vi "Global settings.vi"() -> ()   [LabVIEW 2018]
uses:
  <vilib>/Utility/miscctls.llb/LVDateTimeRec.ctl
  <vilib>/addons/database/Auxilliary.llb/DB Tools Format Datetime String (Time Stamp).vi
  <vilib>/lvdsc/NI_DSC.lvlib
  <vilib>/addons/database/NI_Database_API.lvlib
panel:
  in  "Clear":bool
  out "date time rec 4":T1
  out "x-y 2":T1
  out "Accident 2":bool
  out "Database Data":i32(listbox)=-1
  in  "Accident":bool
  in  "Traffic light failure":bool
  in  "Closesettings":bool
  in  "Set state":T2(ring)
  in  "State change":bool=TRUE
  in  "Time scale":dbl=1.0
  out "date time rec":T1
  out "x > y?":bool
  in  "Difference":dbl=5.0
  in  "Traffic volume 2":dbl(knob) scale=0.0..10.0
  in  "Traffic volume 1":dbl(knob) scale=0.0..10.0
  # "AUTO"
  # "MANUAL"
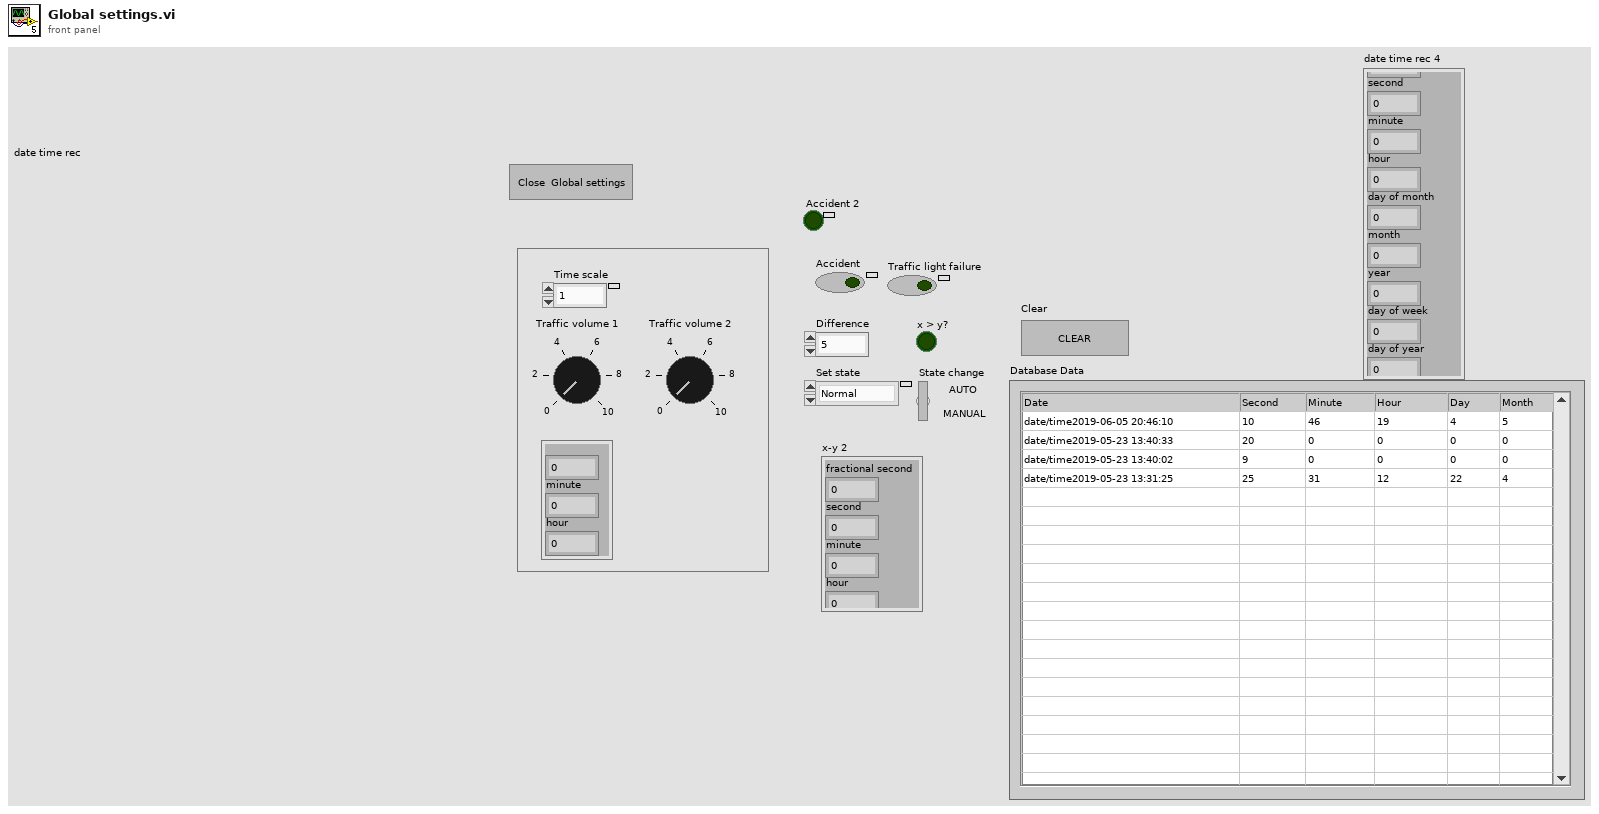
[diagram p1: front panel]
types:
  T1 = typedef "LVDateTimeRec.ctl" = cluster{"fractional second":dbl, "second":i32, "minute":i32, "hour":i32, "day of month":i32, "month":i32, "year":i32, "day of week":i32, "day of year":i32, "DST":i32}
  T2 = enum16{"Normal", "Night", "Traffic jam 1", "Traffic jam 2"}
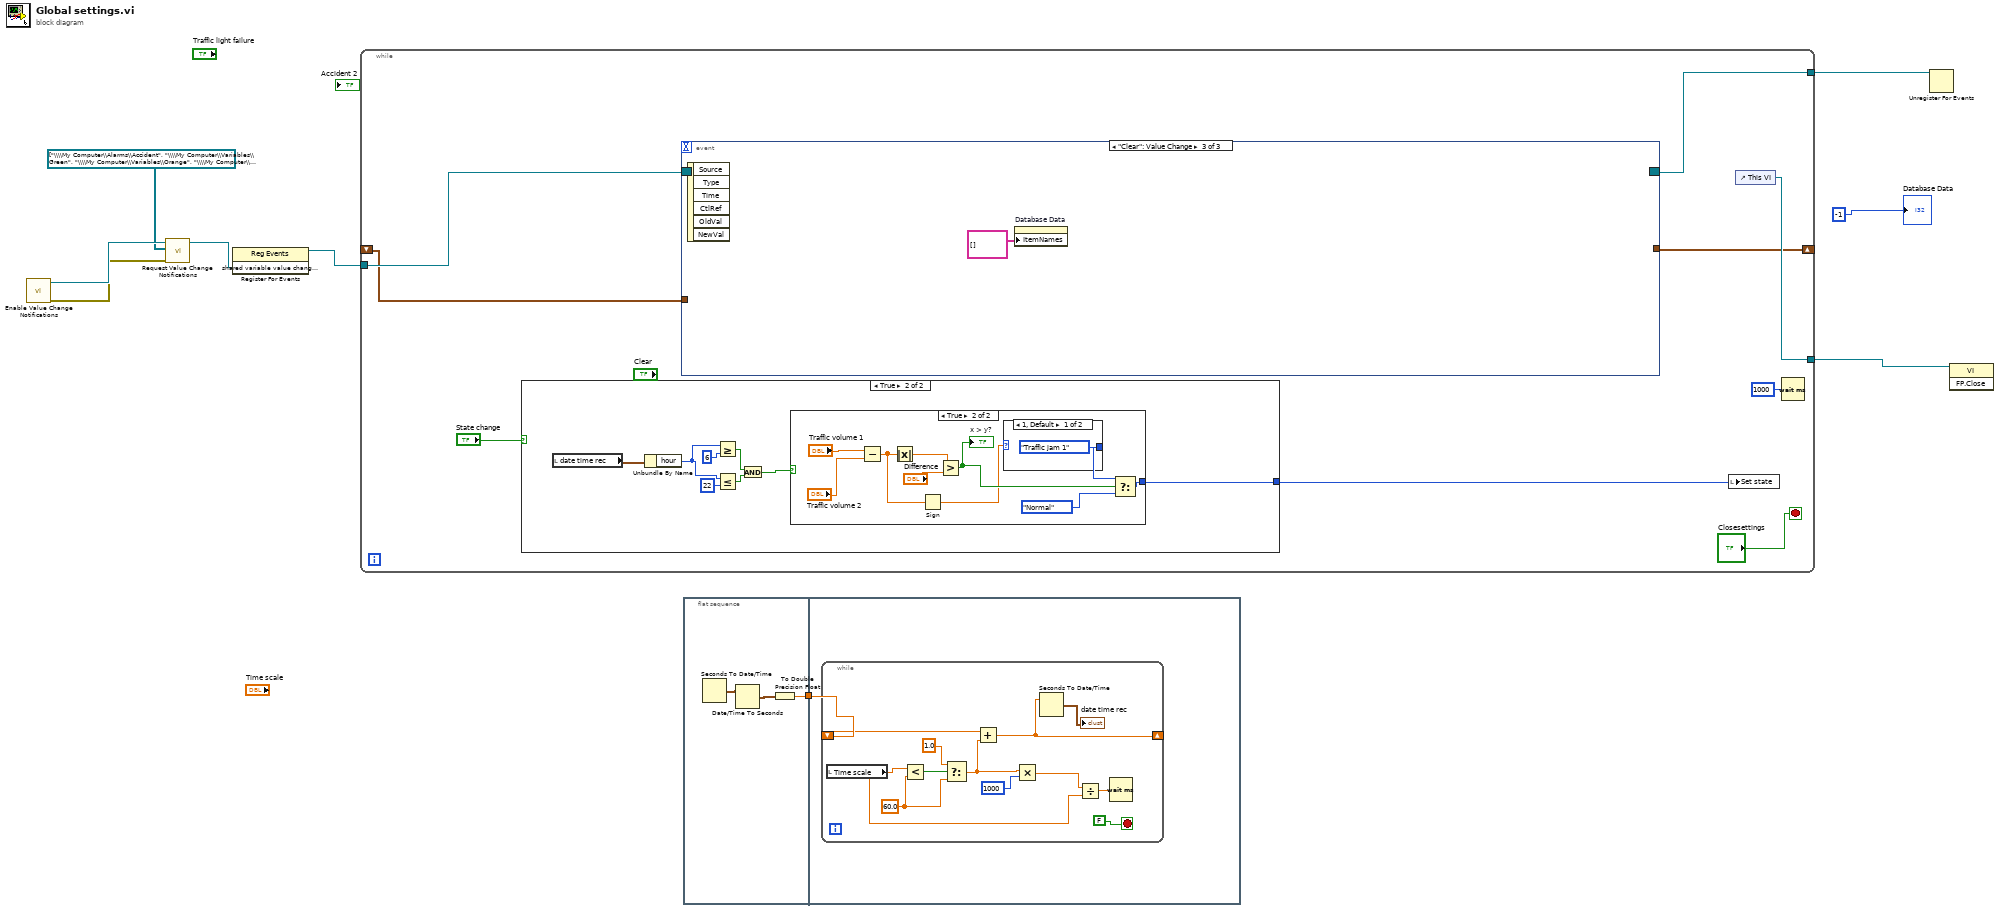
[diagram p0: block diagram]
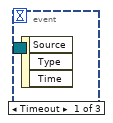
[diagram p2: hidden frame]
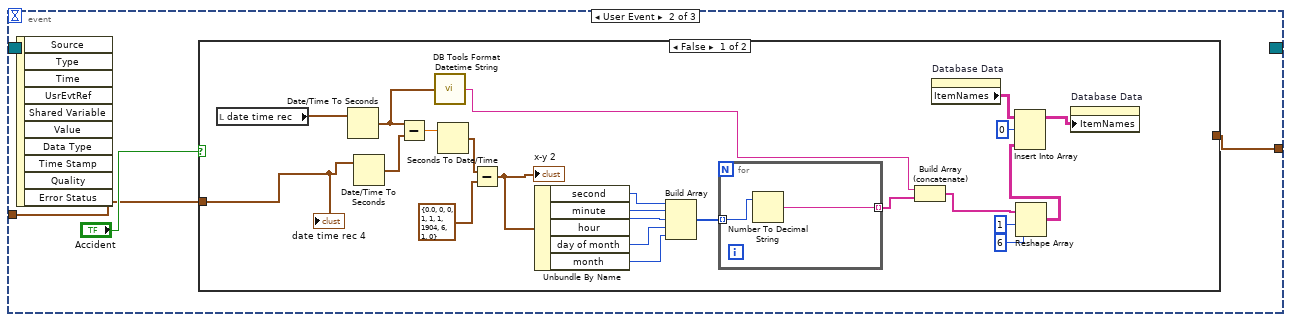
[diagram p3: hidden frame]
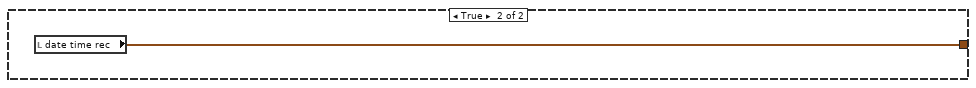
[diagram p4: hidden frame]
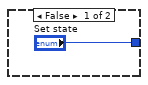
[diagram p5: hidden frame]
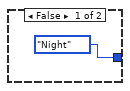
[diagram p6: hidden frame]
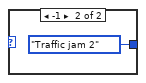
[diagram p7: hidden frame]
diagram:
  n1 = call <vilib>:"Enable Value Change Notifications.vi"() -> ("error out"=w4:errorcluster, "shared variable value change notification"=w5:refnum<user-event>)  [unwired: 1 in, 9 out]
  n2 = call <vilib>:"Request Value Change Notifications.vi"("error in (no error)"=w4, "shared variables"=refnum<k21>[] ["\\\\My Computer\\Alarms\\Accident", "\\\\My Computer\\Variables\\Green", "\\\\My Computer\\Variables\\Orange", "\\\\My Computer\\Variables\\Red", "\\\\My Computer\\Variables\\Yellow"], "notification refnum"=w5) -> ("shared variable value change notification"=w6:refnum<user-event>)  [unwired: 1 in, 7 out]
  n3 = register-events(w6) -> (reference out=w2:refnum<event-registration>)  [unwired: 2 in, 1 out]
  n4 = while {
    tunnel: [w15] -> w8
    tunnel: w2 -> [w13]
    tunnel: [w12] -> w1
    shift-right: [w11] -> _
    shift-left: _ -> [w10]
    stop <- "Closesettings" stop-if-true
    n5 = case shown="True" "State change" {
      tunnel: ["Set state" w50] -> w16
      frame False {
      }
      frame True {
        n6 = local read "date time rec"() -> (w57:T1)
        n7 = Unbundle By Name(w57) -> ("hour"=w51:i32)
        n8 = Greater Or Equal?(x=w51, y=6 ("x")) -> (x >= y?=w56:bool)
        n9 = Less Or Equal?(x=w51, y=22) -> (x <= y?=w54:bool)
        n10 = And(x=w56, y=w54) -> (x .and. y?=w53:bool)
        n11 = case shown="True" w53 {
          tunnel: [T2."Night" ("Set state") w61] -> w50
          frame False {
          }
          frame True {
            n12 = Subtract(x="Traffic volume 1", y="Traffic volume 2") -> (x-y=w63:dbl)
            n13 = Absolute Value(x=w63) -> (abs(x)=w66:dbl)
            n14 = Sign(1:w63) -> (0:w60:dbl)
            n15 = Greater?(x=w66, y="Difference") -> (0:w64:bool)
            "x > y?" <- w64
            n16 = case shown="1, Default" w60 {
              tunnel: [T2."Traffic jam 1" ("Set state") T2."Traffic jam 2" ("Set state")] -> w59
              frame 1, Default {
              }
              frame -1 {
              }
            }
            n17 = Select(t=w59, s=w64, f=T2."Normal" ("Set state")) -> (s? t:f=w61:T2)
          }
        }
      }
    }
    n18 = event shown="[2] \"Clear\": Value Change" {
      selector: w13 -> [_ _ _]
      dyn-events: [_ _ _] -> w12
      timeout: _ -> [_ _ _]
      tunnel: [_ w20 _] -> w11
      tunnel: w10 -> [_ w19 _]
      event Timeout {
        n19 = event-data() -> ()  [unwired: 1 in, 3 out]
      }
      event User Event {
        n20 = event-data() -> ()  [unwired: 1 in, 10 out]
        n21 = case shown="False" "Accident" {
          tunnel: [_ w47] -> w20
          tunnel: w19 -> [w39 _]
          frame False {
            n22 = local read "date time rec"() -> (w44:T1)
            n23 = Date/Time To Seconds(2:w44) -> (0:w25:timestamp)  [unwired: 1 in]
            n24 = Date/Time To Seconds(2:w39) -> (0:w43:timestamp)  [unwired: 1 in]
            n25 = Subtract(x=w25, y=w43) -> (x-y=w42:dbl)
            n26 = call-poly <vilib>:"DB Tools Format Datetime String.vi"("time stamp"=w25) -> ("date/time string"=w22:string)
            n27 = Seconds To Date/Time(time stamp (now)=w42) -> (date time rec=w41:T1)  [unwired: 1 in]
            n28 = Subtract(x=w41, y=T1 {"fractional second"=0.0, "second"=0, "minute"=0, "hour"=1, "day of month"=1, "month"=1, "year"=1904, "day of week"=6, "day of year"=1, "DST"=0} ("date time rec")) -> (x-y=w33:T1)
            "x-y 2" <- w33
            n29 = Unbundle By Name(w33) -> ("second"=w38:i32, "minute"=w37:i32, "hour"=w36:i32, "day of month"=w35:i32, "month"=w34:i32)
            n30 = Build Array(w38, w37, w36, w35, w34) -> (w32:i32[])
            n31 = for {
              tunnel: w32 -> [w46] mode=indexing
              tunnel: [w45] -> w24 mode=indexing
              n32 = Number To Decimal String(number=w46) -> (decimal integer string=w45:string)  [unwired: 1 in]
            }
            n33 = Build Array (concatenate)(w22, w24) -> (w23:string[])
            n34 = property on="Database Data" class="MCListbox (strict)"() -> ("ItemNames"=w29:string[][])  [unwired: 2 in, 2 out]
            n35 = Reshape Array "Reshape Array"(w23, 1 ("dimension size"), 6 ("dimension size")) -> (w28:string[][])
            n36 = Insert Into Array(array=w29, index (row)=0, new element=w28) -> (w27:string[][])  [unwired: 1 in]
            n37 = property on="Database Data" class="MCListbox (strict)"("ItemNames"=w27) -> ()  [unwired: 2 in, 2 out]
            "date time rec 4" <- w39
          }
          frame True {
            n38 = local read "date time rec"() -> (w47:T1)
          }
        }
      }
      event "Clear": Value Change {
        n39 = event-data() -> ()  [unwired: 1 in, 6 out]
        n40 = property on="Database Data" class="MCListbox (strict)"("ItemNames"=string[][] [] ("Item Names")) -> ()  [unwired: 2 in, 2 out]
      }
    }
    n41 = local write "Set state"(w16) -> ()
    n42 = control-ref of="This VI"() -> (w15:refnum<vi>)
    n43 = Wait (ms)(milliseconds to wait=u32 1000) -> ()  [unwired: 1 out]
  }
  n44 = flat-sequence {
    tunnel: [w71] -> w9
    tunnel: w9 -> [w74]
    frame #0 {
      n45 = Seconds To Date/Time() -> (date time rec=w73:T1)  [unwired: 2 in]
      n46 = Date/Time To Seconds(2:w73) -> (0:w72:timestamp)  [unwired: 1 in]
      n47 = To Double Precision Float(number=w72) -> (double precision float=w71:dbl)
    }
    frame #1 {
      n48 = while {
        shift-right: [w83] -> _
        shift-left: w74 -> [w84]
        stop <- FALSE stop-if-true
        w78 = 60.0 ("f")
        n49 = local read "Time scale"() -> (w79:dbl)
        n50 = Less?(x=w79, y=w78) -> (x < y?=w80:bool)
        n51 = Select(t=1.0, s=w80, f=w78) -> (s? t:f=w76:dbl)
        n52 = Add(x=w84, y=w76) -> (x+y=w83:dbl)
        n53 = Multiply(x=w76, y=u32 1000 ("milliseconds to wait")) -> (x*y=w75:dbl)
        n54 = Seconds To Date/Time(time stamp (now)=w83) -> (date time rec=→"date time rec":T1)  [unwired: 1 in]
        n55 = Divide(x=w75, y=w79) -> (x/y=w82:dbl)
        n56 = Wait (ms)(milliseconds to wait=w82) -> ()  [unwired: 1 out]
      }
    }
  }
  n57 = Unregister For Events(event registration refnum=w1) -> ()  [unwired: 1 in, 1 out]
  n58 = invoke class="VI" method="FP.Close"(reference=w8) -> ()  [unwired: 2 in, 3 out]
  "Database Data" <- -1 ("Database Data")
